vi "SQLite Delete Category Test.vi"(7 "Test DB Set Up Command":string, 8 "Error In (no error)":errorcluster, 11 "SQLite DB Operator In":refnum<class "SQLite DB Operator.lvclass">) -> (0 "Error Out":errorcluster, 3 "SQLite DB OperatorOut":refnum<class "SQLite DB Operator.lvclass">)   [LabVIEW 2023]
uses:
  Clasess/SQLite DB Operator/SQLite DB Operator.lvclass
  Clasess/DB Records/Expenses Tracker Category/Public/Ctrls/Category.ctl
  Clasess/DB Records/Expenses Tracker Category/Expenses Tracker Category.lvclass
  H:/Desktop/LabVIEW/LabView Repo/Expenses-Tracker-DB-Operator/Interfaces/Expenses Tracker Record/Expenses Tracker Record.lvclass
  Support/Editing/Edit Record Assert Error.vi
  Support/Editing/Edit Record Assert Not Error.vi
  <vilib>/drjdpowell/SQLite Library/SQL Connection/Execute SQL (1D Cluster).vi
  <vilib>/addons/_JKI Toolkits/Caraya/classes/Test/Test.lvclass
  <vilib>/drjdpowell/SQLite Library/SQLite.lvlib
  H:/Desktop/LabVIEW/LabView Repo/Expenses-Tracker-DB-Operator/Clasess/DB Records/Expenses Tracker Category/Expenses Tracker Category.lvclass
  <vilib>/drjdpowell/SQLite Library/SQL Connection/Connection.lvclass
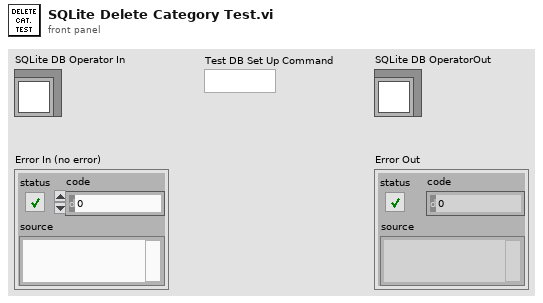
[diagram p1: front panel]
types:
  T1 = typedef "Expenses Tracker Category.lvclass/Category.ctl" = cluster{"ID":u32, "Name":string}
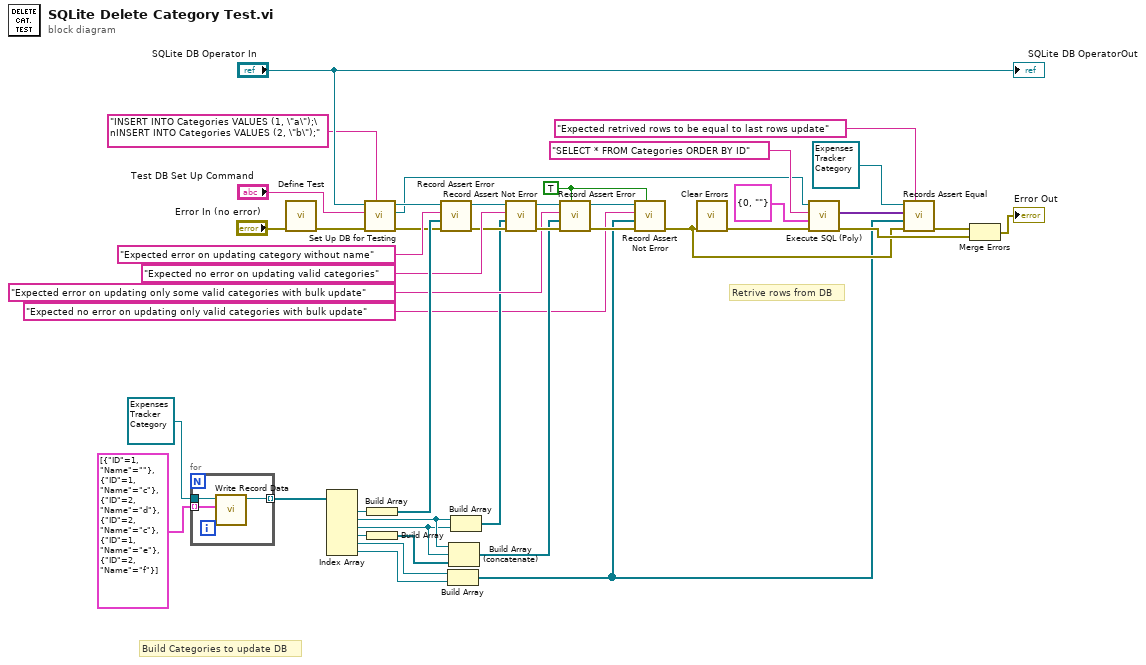
[diagram p0: block diagram]
diagram:
  w10 = TRUE ("Bulk Insert?")
  # "Retrive rows from DB"
  # "Build Categories to update DB"
  n1 = for {
    tunnel: T1[] [{"ID"=1, "Name"=""}, {"ID"=1, "Name"="c"}, {"ID"=2, "Name"="d"}, {"ID"=2, "Name"="c"}, {"ID"=1, "Name"="e"}, {"ID"=2, "Name"="f"}] ("Array") -> [w46] mode=indexing
    tunnel: refnum<class "Expenses Tracker Category.lvclass"> refnum ("Expenses Tracker Category") -> [w45]
    tunnel: [w44] -> w40 mode=indexing
    n2 = call-dynamic "Write Record Data.vi"("Record"=w46, "Expenses Tracker Category In"=w45) -> ("Expenses Tracker Category Out"=w44:refnum<class "Expenses Tracker Category.lvclass">)  [unwired: 8 in, 1 out]
  }
  n3 = call <vilib>:"Define Test.vi"("error in (no error)"="Error In (no error)") -> ("error out"=w29:errorcluster)  [unwired: 9 in, 1 out]
  n4 = Index Array(array=w40) -> (element #1=w39:refnum<class "Expenses Tracker Category.lvclass">, element #2=w18:refnum<class "Expenses Tracker Category.lvclass">, element #3=w17:refnum<class "Expenses Tracker Category.lvclass">, element #4=w37:refnum<class "Expenses Tracker Category.lvclass">, element #5=w4:refnum<class "Expenses Tracker Category.lvclass">, element #6=w3:refnum<class "Expenses Tracker Category.lvclass">)  [unwired: 6 in]
  n5 = call "Set Up DB for Testing.vi"("Additional Set Up Commands"="INSERT INTO Categories VALUES (1, \"a\");\nINSERT INTO Categories VALUES (2, \"b\");", "Error In (no error)"=w29, "Test DB Set Up Command"="Test DB Set Up Command", "SQLite DB Operator In"="SQLite DB Operator In") -> ("Error Out"=w28:errorcluster, "SQLite Connection"=w31:refnum<class "Connection.lvclass">, "SQLite DB Operator Out"=w33:refnum<class "SQLite DB Operator.lvclass">)  [unwired: 5 in]
  n6 = Build Array(w39) -> (w38:refnum<class "Expenses Tracker Category.lvclass">[])
  n7 = Build Array(w37) -> (w16:refnum<class "Expenses Tracker Category.lvclass">[])
  n8 = call-poly "Record Assert Error.vi"("Error In"=w28, "Records"=w38, "Assertion Label"="Expected error on updating category without name" ("Label (VI Title)"), "SQLite DB Operator In"=w33) -> ("Error Out"=w25:errorcluster, "SQLite DB Operator Out"=w27:refnum<class "SQLite DB Operator.lvclass">)  [unwired: 6 in]
  n9 = Build Array(w4, w3) -> (w2:refnum<class "Expenses Tracker Category.lvclass">[])
  n10 = Build Array (concatenate)(w18, w17, w16) -> (w12:refnum<class "Expenses Tracker Category.lvclass">[])
  n11 = Build Array(w18, w17) -> (w6:refnum<class "Expenses Tracker Category.lvclass">[])
  n12 = call-poly "Record Assert Not Error.vi"("Error In"=w25, "Records"=w6, "Assertion Label"="Expected no error on updating valid categories" ("Label (VI Title)"), "SQLite DB Operator In"=w27) -> ("Error Out"=w15:errorcluster, "SQLite DB Operator Out"=w14:refnum<class "SQLite DB Operator.lvclass">)  [unwired: 6 in]
  n13 = call-poly "Record Assert Error.vi"("Bulk Update?"=w10, "Error In"=w15, "Records"=w12, "Assertion Label"="Expected error on updating only some valid categories with bulk update" ("Label (VI Title)"), "SQLite DB Operator In"=w14) -> ("Error Out"=w8:errorcluster, "SQLite DB Operator Out"=w9:refnum<class "SQLite DB Operator.lvclass">)  [unwired: 5 in]
  n14 = call-poly "Record Assert Not Error.vi"("Bulk Update?"=w10, "Error In"=w8, "Records"=w2, "Assertion Label"="Expected no error on updating only valid categories with bulk update" ("Label (VI Title)"), "SQLite DB Operator In"=w9) -> ("Error Out"=w7:errorcluster)  [unwired: 5 in, 1 out]
  n15 = call <vilib>:"Clear Errors.vi"("error in (no error)"=w7) -> ("error out"=w23:errorcluster)  [unwired: 5 in, 1 out]
  n16 = call-poly <vilib>:"Execute SQL (Poly).vi"("error in (no error)"=w23, "Cluster (or Array of Clusters)"=T1 {"ID"=0, "Name"=""} ("Category"), "SQL"="SELECT * FROM Categories ORDER BY ID", "SQLite Connection in"=w31) -> ("error out"=w20:errorcluster, "Result Set (Array of Clusters)"=w1:variant[])  [unwired: 5 in, 1 out]
  n17 = call "Records Assert Equal.vi"("Assertion Label"="Expected retrived rows to be equal to last rows update" ("Label (VI Title)"), "Error In"=w7, "Correct Records"=w2, "Typedef Records"=w1, "Expenses Tracker Record In"=refnum<class "Expenses Tracker Category.lvclass"> refnum ("Expenses Tracker Category")) -> ("Error Out"=w34:errorcluster)  [unwired: 6 in]
  n18 = Merge Errors(w34, w20) -> (→"Error Out":errorcluster)
  "SQLite DB OperatorOut" <- "SQLite DB Operator In"
